vi "file list - accumulate paths.vi"(11 "file path":path=path "/snowfall/Users/arcadi/Desktop/Ultrasound/Experiment/YBCO_4/Round1/Sweep12/June_2011/062511/221.16400K_300_3100_001_062511.dat") -> (0 "Array OUT":path[](array[path]))   [LabVIEW 2010]
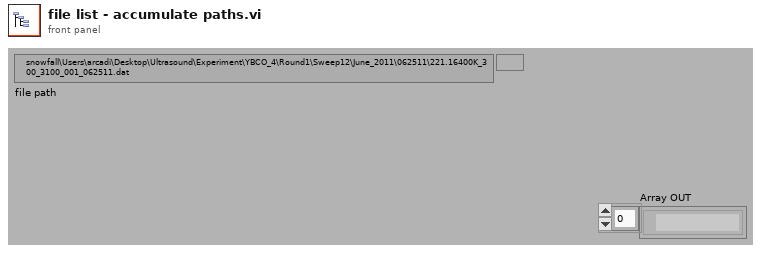
[diagram p1: front panel]
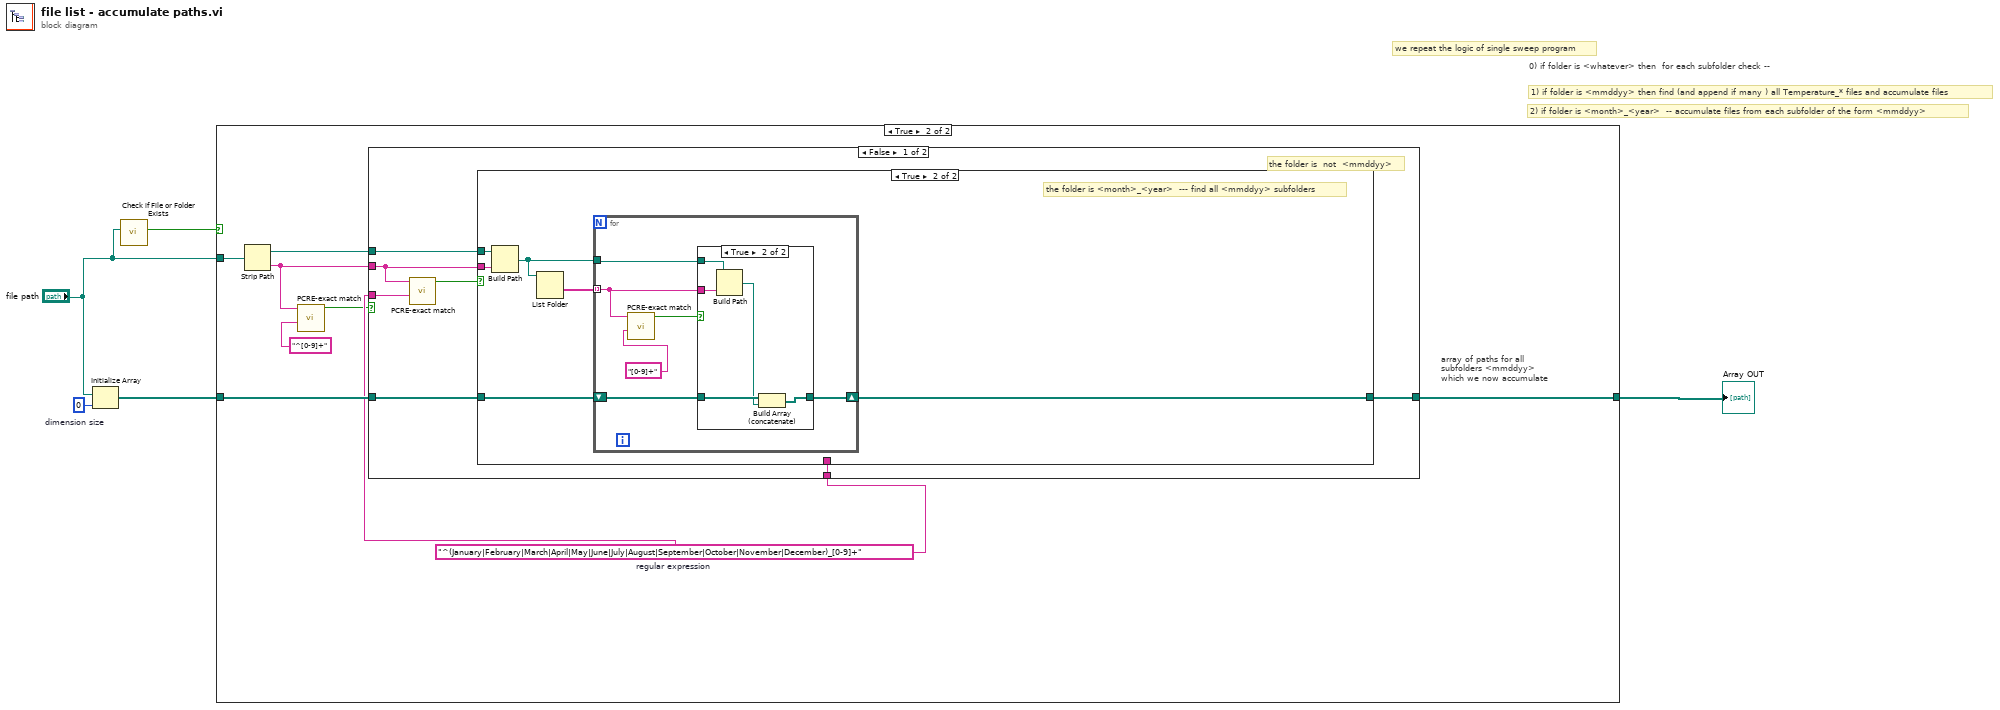
[diagram p0: block diagram]
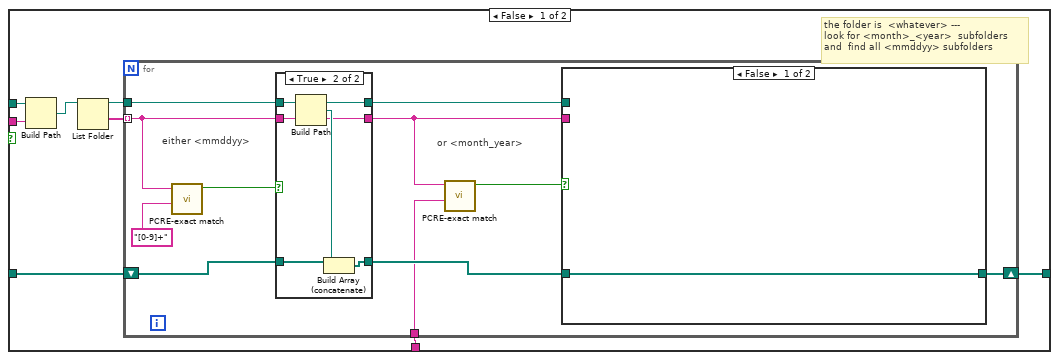
[diagram p3: hidden frame]
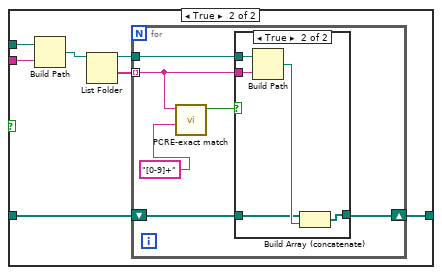
[diagram p4: hidden frame]
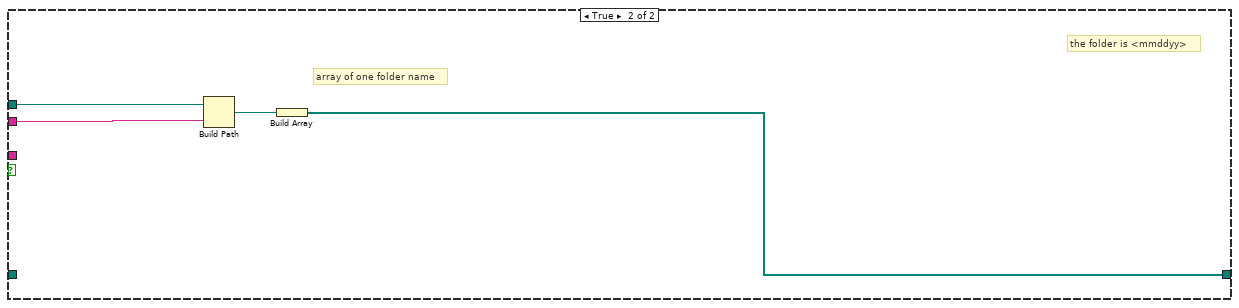
[diagram p8: hidden frame]
diagram:
  w4 = 0  # dimension size
  # "0) if folder is <whatever> then  for each subfolder check --"
  # "1) if folder is <mmddyy> then find (and append if many ) all Temperature_* files and accumulate files"
  # "2) if folder is <month>_<year>  -- accumulate files from each subfolder of the form <mmddyy>"
  # "we repeat the logic of single sweep program"
  n1 = Initialize Array("file path", w4) -> (w2:path[])
  n2 = call <vilib>:"Check if File or Folder Exists.vi"("path"="file path") -> ("file or folder exists?"=w5:bool)  [unwired: 8 in, 2 out]
  n3 = case shown="True" w5 {
    tunnel: "file path" -> [_ w14]
    tunnel: w2 -> [w6 w12]
    tunnel: [w6 w7] -> w1
    frame False {
    }
    frame True {
      w11 = "^(January|February|March|April|May|June|July|August|September|October|November|December)_[0-9]+"  # regular expression
      # "array of paths for all  \nsubfolders <mmddyy>\nwhich we now accumulate"
      n4 = Strip Path(path=w14) -> (stripped path=w13:path, name=w10:string)
      n5 = call "PCRE-exact match.vi"("regular expression"="^[0-9]+", "input string"=w10) -> ("exact match"=w8:bool)  [unwired: 8 in, 1 out]
      n6 = case shown="False" w8 {
        tunnel: [w21 w89] -> w7
        tunnel: w13 -> [w20 w88]
        tunnel: w10 -> [w16 w87]
        tunnel: w11 -> [w17 _]
        tunnel: w12 -> [w19 _]
        tunnel: w11 -> [w18 _]
        frame False {
          # "the folder is  not  <mmddyy>"
          n7 = call "PCRE-exact match.vi"("regular expression"=w17, "input string"=w16) -> ("exact match"=w15:bool)  [unwired: 8 in, 1 out]
          n8 = case shown="True" w15 {
            tunnel: [w23 w72] -> w21
            tunnel: w16 -> [w26 w71]
            tunnel: w20 -> [w27 w70]
            tunnel: w19 -> [w25 w69]
            tunnel: w18 -> [w24 _]
            frame False {
              # "the folder is  <whatever> --- \nlook for <month>_<year>  subfolders \nand  find all <mmddyy> subfolders"
              n9 = Build Path(base path=w27, name or relative path=w26) -> (appended path=w28:path)
              n10 = List Folder(path=w28) -> (path out=w22:path, folder names=w29:string[])  [unwired: 3 in, 2 out]
              n11 = for {
                tunnel: w29 -> [w35] mode=indexing
                shift-right: [w39] -> w23
                shift-left: w25 -> [w40]
                tunnel: w22 -> [w37]
                tunnel: w24 -> [w31]
                # "or <month_year>"
                # "either <mmddyy>"
                n12 = call "PCRE-exact match.vi"("regular expression"="[0-9]+", "input string"=w35) -> ("exact match"=w33:bool)  [unwired: 8 in, 1 out]
                n13 = case shown="True" w33 {
                  tunnel: w37 -> [w61 w64]
                  tunnel: w35 -> [w62 w65]
                  tunnel: w40 -> [w63 w68]
                  tunnel: [w63 w66] -> w38
                  tunnel: [w62 w65] -> w32
                  tunnel: [w61 w64] -> w36
                  frame False {
                  }
                  frame True {
                    n14 = Build Path(base path=w64, name or relative path=w65) -> (appended path=w67:path)
                    n15 = Build Array (concatenate)(w68, w67) -> (w66:path[])
                  }
                }
                n16 = call "PCRE-exact match.vi"("regular expression"=w31, "input string"=w32) -> ("exact match"=w30:bool)  [unwired: 8 in, 1 out]
                n17 = case shown="False" w30 {
                  tunnel: [w41 w44] -> w39
                  tunnel: w38 -> [w41 w45]
                  tunnel: w36 -> [_ w48]
                  tunnel: w32 -> [_ w47]
                  frame False {
                  }
                  frame True {
                    n18 = Build Path(base path=w48, name or relative path=w47) -> (appended path=w43:path)
                    n19 = List Folder(path=w43) -> (path out=w42:path, folder names=w46:string[])  [unwired: 3 in, 2 out]
                    n20 = for {
                      tunnel: w46 -> [w51] mode=indexing
                      shift-right: [w53] -> w44
                      shift-left: w45 -> [w54]
                      tunnel: w42 -> [w52]
                      n21 = call "PCRE-exact match.vi"("regular expression"="[0-9]+", "input string"=w51) -> ("exact match"=w49:bool)  [unwired: 8 in, 1 out]
                      n22 = case shown="True" w49 {
                        tunnel: w54 -> [w55 w59]
                        tunnel: [w55 w58] -> w53
                        tunnel: w52 -> [_ w57]
                        tunnel: w51 -> [_ w56]
                        frame False {
                        }
                        frame True {
                          n23 = Build Path(base path=w57, name or relative path=w56) -> (appended path=w60:path)
                          n24 = Build Array (concatenate)(w59, w60) -> (w58:path[])
                        }
                      }
                    }
                  }
                }
              }
            }
            frame True {
              # "the folder is <month>_<year>  --- find all <mmddyy> subfolders"
              n25 = Build Path(base path=w70, name or relative path=w71) -> (appended path=w73:path)
              n26 = List Folder(path=w73) -> (folder names=w74:string[])  [unwired: 3 in, 3 out]
              n27 = for {
                tunnel: w74 -> [w77] mode=indexing
                shift-right: [w78] -> w72
                shift-left: w69 -> [w79]
                tunnel: w73 -> [w80]
                n28 = call "PCRE-exact match.vi"("regular expression"="[0-9]+", "input string"=w77) -> ("exact match"=w75:bool)  [unwired: 8 in, 1 out]
                n29 = case shown="True" w75 {
                  tunnel: w80 -> [_ w86]
                  tunnel: w77 -> [_ w85]
                  tunnel: w79 -> [w81 w84]
                  tunnel: [w81 w82] -> w78
                  frame False {
                  }
                  frame True {
                    n30 = Build Path(base path=w86, name or relative path=w85) -> (appended path=w83:path)
                    n31 = Build Array (concatenate)(w84, w83) -> (w82:path[])
                  }
                }
              }
            }
          }
        }
        frame True {
          # "the folder is <mmddyy>"
          # "array of one folder name"
          n32 = Build Path(base path=w88, name or relative path=w87) -> (appended path=w90:path)
          n33 = Build Array(w90) -> (w89:path[])
        }
      }
    }
  }
  "Array OUT" <- w1
